vi "Tool num2OKNG.vi"(11 "1:OK/ 2:NG":i16) -> (3 "檢測結果":string)   [LabVIEW 2019]
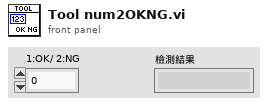
[diagram p1: front panel]
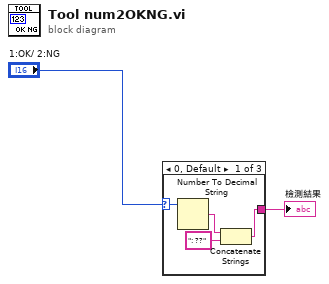
[diagram p0: block diagram]
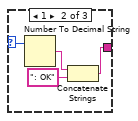
[diagram p2: hidden frame]
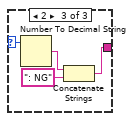
[diagram p3: hidden frame]
diagram:
  n1 = case shown="0, Default" "1:OK/ 2:NG" {
    selector: "1:OK/ 2:NG" -> [w4 w8 w14]
    tunnel: [w3 w7 w11] -> w2
    frame 0, Default {
      n2 = Number To Decimal String(number=w4) -> (decimal integer string=w6:string)  [unwired: 1 in]
      n3 = Concatenate Strings(w6, ": ??" ("string")) -> (w3:string)
    }
    frame 1 {
      n4 = Number To Decimal String(number=w8) -> (decimal integer string=w10:string)  [unwired: 1 in]
      n5 = Concatenate Strings(w10, ": OK" ("string")) -> (w7:string)
    }
    frame 2 {
      n6 = Number To Decimal String(number=w14) -> (decimal integer string=w13:string)  [unwired: 1 in]
      n7 = Concatenate Strings(w13, ": NG" ("string")) -> (w11:string)
    }
  }
  "檢測結果" <- w2
